vi "Write State.vi"(8 "error in (no error)":errorcluster, 10 "State":u16, 11 "AutoExp in":refnum<class "AutoExp.lvclass">) -> (0 "error out":errorcluster, 3 "AutoExp out":refnum<class "AutoExp.lvclass">)   [LabVIEW 2018, in "AutoExp.lvclass"]
uses:
  AutoExp.lvclass
  AutoExp.lvclass/AutoExp.ctl
  State Machine/State Machine.lvclass
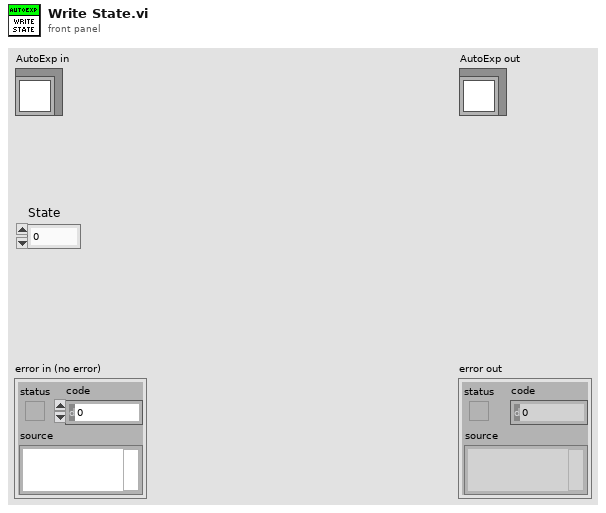
[diagram p1: front panel]
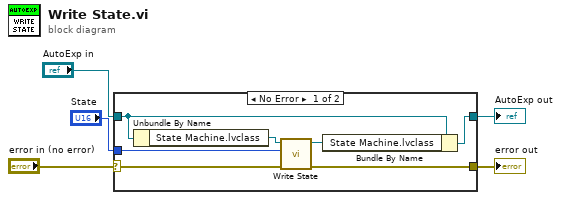
[diagram p0: block diagram]
diagram:
  n1 = case shown="No Error" "error in (no error)" {
    selector: "error in (no error)" -> [w12 w14]
    tunnel: [w11 w14] -> w4
    tunnel: [w10 w13] -> w2
    tunnel: "AutoExp in" -> [w9 w13]
    tunnel: "State" -> [w6 _]
    frame No Error {
      n2 = Unbundle By Name(w9) -> ("State Machine.lvclass"=w7:refnum<class "State Machine.lvclass">)
      n3 = call-dynamic "Write State.vi"("error in (no error)"=w12, "State"=w6, "State Machine in"=w7) -> ("error out"=w11:errorcluster, "State Machine out"=w8:refnum<class "State Machine.lvclass">)  [unwired: 7 in]
      n4 = Bundle By Name(cluster=w9, "State Machine.lvclass"=w8) -> (w10:refnum<class "AutoExp.lvclass">)
    }
    frame Error {
    }
  }
  "error out" <- w4
  "AutoExp out" <- w2
